vi "Actor Core.vi"(8 "error in":errorcluster, 11 "Assert Display in":refnum<class "Assert Display.lvclass">) -> (0 "error out":errorcluster, 3 "Actor out":refnum<class "Actor.lvclass">)   [LabVIEW 2016, in "Assert Display.lvlib" / "Assert Display.lvclass"]
doc: "(<B>Filename</B>: Actor Framework.lvlib:Actor.lvclass:Actor Core.vi)\n\nReceives messages to the actor, reacts to them, and initiates any error handling that may shut the actor down.\n\nDescendant classes may override this VI to append parallel tasks for the actor to complete while it handles messages. Overrides use the Call Parent Method node."
uses:
  Assert Display.lvclass
  C:/Program Files (x86)/National Instruments/LabVIEW 2016/vi.lib/ActorFramework/Actor/Actor.lvclass
  D:/Work/Projects/Actor_Assert_API/Base UI Actor/Base UI Actor/Base UI Actor.lvclass
  <vilib>/ActorFramework/Actor/Actor.lvclass
  Filter Config Display/Filter Config Display/Filter Config Display.lvclass
  D:/Work/Projects/Actor_Assert_API/Base UI Component/Base UI Component/Base UI Component.lvclass
  Main Display/Main Display/Main Display.lvclass
  Service Config Display/Service Config Display/Service Config Display.lvclass
  Base UI Actor/Base UI Actor/Base UI Actor.lvclass/Base UI Actor.ctl
  <vilib>/ActorFramework/Actor/Actor.lvclass/Actor.ctl
  <vilib>/ActorFramework/Message Enqueuer/Message Enqueuer.lvclass/Message Enqueuer.ctl
  Assert Display.lvclass/Assert Display.ctl
  Assert Display Messages/Change Screen Msg/Change Screen Msg.lvclass/Change Screen Msg.ctl
  <vilib>/ActorFramework/Message Enqueuer/Init from Existing Queue.vi
  <vilib>/ActorFramework/Message Enqueuer/Enqueue.vi
  <vilib>/ActorFramework/Stop Msg/Stop Msg.lvclass
  C:/Program Files (x86)/National Instruments/LabVIEW 2016/vi.lib/ActorFramework/Message/Message.lvclass
  Assert Display Messages/Change Screen Msg/Change Screen Msg.lvclass
  <vilib>/ActorFramework/Message Priority Queue/Priority Enqueue.vi
  <vilib>/ActorFramework/Message Enqueuer/Message Enqueuer.lvclass
  Base UI Actor/Base UI Actor/Base UI Actor.lvclass
  Base UI Component/Base UI Component/Base UI Component.lvclass
panel:
  in  "Filters":bool
  in  "Services":bool
  in  "Main":bool
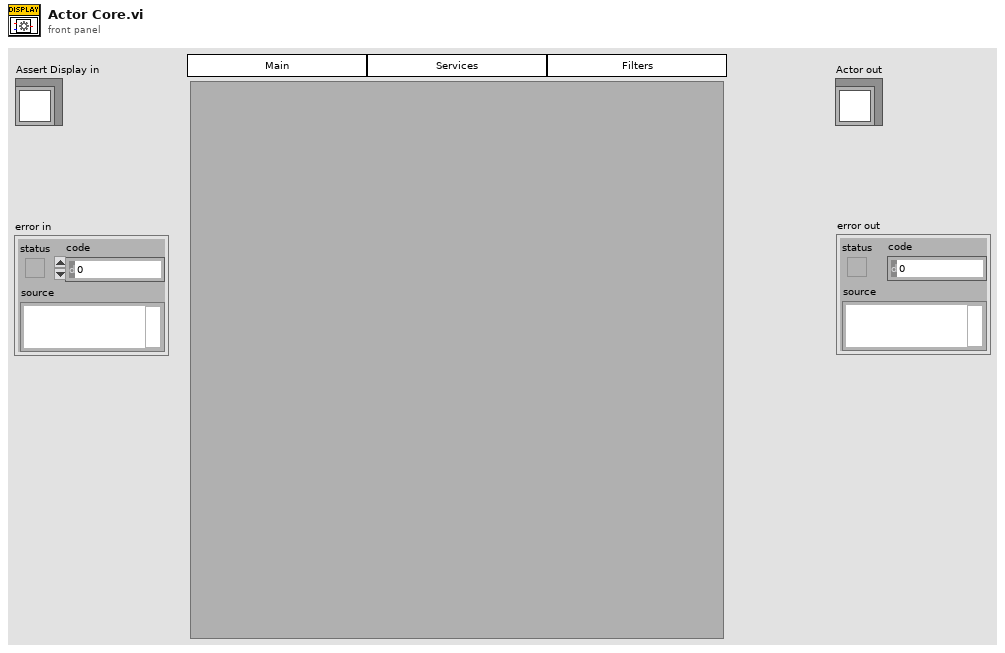
[diagram p1: front panel]
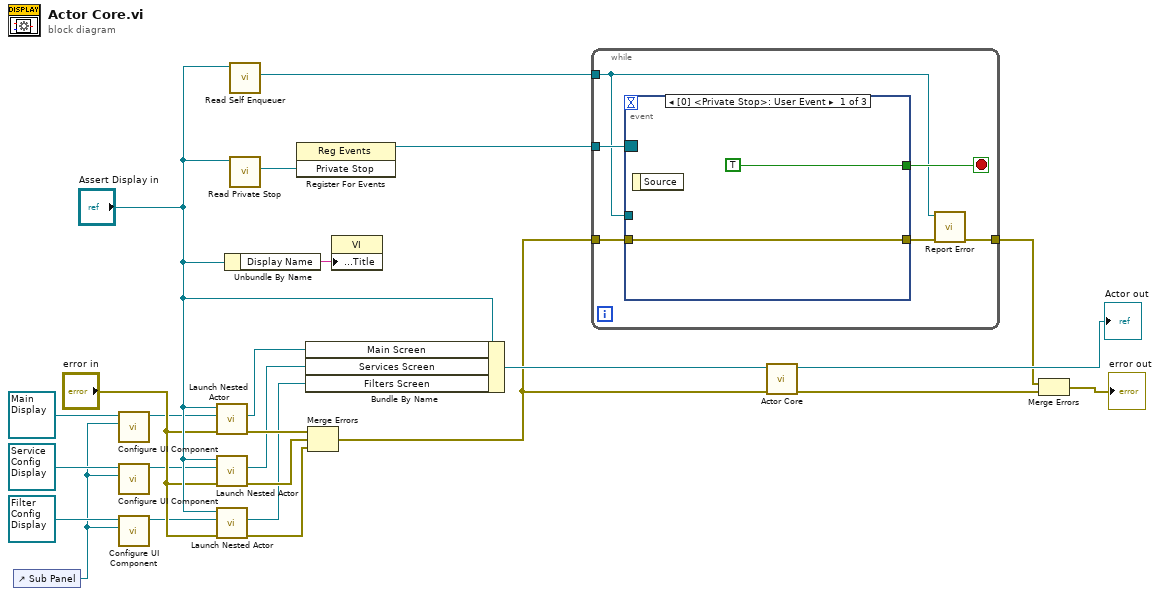
[diagram p0: block diagram]
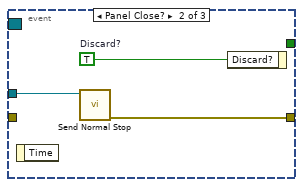
[diagram p2: hidden frame]
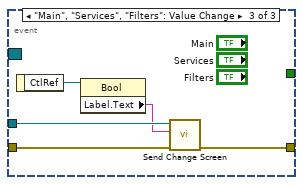
[diagram p3: hidden frame]
diagram:
  n1 = control-ref of="Sub Panel"() -> (w1:refnum<vi>)
  n2 = call "Configure UI Component.vi"("SubPanel Reference"=w1, "Base UI Component in"=refnum<class "Main Display.lvclass"> refnum ("Assert Display.lvlib:Main Display.lvlib:Main Display.lvclass")) -> ("Base UI Component out"=w4:refnum<class "Main Display.lvclass">)  [unwired: 9 in]
  n3 = call "Configure UI Component.vi"("SubPanel Reference"=w1, "Base UI Component in"=refnum<class "Service Config Display.lvclass"> refnum ("Assert Display.lvlib:Service Config Display.lvlib:Service Config Display.lvclass")) -> ("Base UI Component out"=w3:refnum<class "Service Config Display.lvclass">)  [unwired: 9 in]
  n4 = call "Configure UI Component.vi"("SubPanel Reference"=w1, "Base UI Component in"=refnum<class "Filter Config Display.lvclass"> refnum ("Assert Display.lvlib:Filter Config Display.lvlib:Filter Config Display.lvclass")) -> ("Base UI Component out"=w2:refnum<class "Filter Config Display.lvclass">)  [unwired: 9 in]
  n5 = call <vilib>:"Launch Nested Actor.vi"("error in (no error)"="error in", "Nested Actor"=w4, "Caller Actor in"="Assert Display in") -> ("error out"=w14:errorcluster, "Nested Actor's Enqueuer"=w10:refnum<class "Message Enqueuer.lvclass">)  [unwired: 6 in, 1 out]
  n6 = call <vilib>:"Launch Nested Actor.vi"("error in (no error)"="error in", "Nested Actor"=w3, "Caller Actor in"="Assert Display in") -> ("error out"=w13:errorcluster, "Nested Actor's Enqueuer"=w9:refnum<class "Message Enqueuer.lvclass">)  [unwired: 6 in, 1 out]
  n7 = call <vilib>:"Launch Nested Actor.vi"("error in (no error)"="error in", "Nested Actor"=w2, "Caller Actor in"="Assert Display in") -> ("error out"=w12:errorcluster, "Nested Actor's Enqueuer"=w8:refnum<class "Message Enqueuer.lvclass">)  [unwired: 6 in, 1 out]
  n8 = Unbundle By Name("Assert Display in") -> ("Display Name"=w23:string)
  n9 = call <vilib>:"Read Self Enqueuer.vi"("Actor"="Assert Display in") -> ("Self Enqueuer"=w20:refnum<class "Message Enqueuer.lvclass">)  [unwired: 10 in]
  n10 = call "Read Private Stop.vi"("Base UI Actor in"="Assert Display in") -> ("Private Stop"=w22:refnum<user-event>)  [unwired: 10 in]
  n11 = register-events(w22) -> (reference out=w21:refnum<event-registration>)  [unwired: 2 in, 1 out]
  n12 = Bundle By Name(cluster="Assert Display in", "Main Screen"=w10, "Services Screen"=w9, "Filters Screen"=w8) -> (w11:refnum<class "Assert Display.lvclass">)
  n13 = Merge Errors(w14, w13, w12) -> (w7:errorcluster)
  n14 = property class="VI"("Front Panel.Title"=w23) -> ()  [unwired: 2 in, 2 out]
  n15 = while {
    tunnel: w21 -> [w31]
    tunnel: w20 -> [w26]
    tunnel: w7 -> [w29]
    tunnel: [w27] -> w5
    stop <- w30 stop-if-true
    n16 = event shown="[0] <Private Stop>: User Event" {
      selector: w31 -> [_ _ _]
      dyn-events: _ -> [_ _ _]
      timeout: _ -> [_ _ _]
      tunnel: [TRUE _ _] -> w30
      tunnel: w26 -> [_ w35 w41]
      tunnel: w29 -> [w32 _ w38]
      tunnel: [w32 w34 w37] -> w28
      event User Event {
        n17 = event-data() -> ()  [unwired: 1 in, 1 out]
      }
      event Panel Close? {
        w36 = TRUE  # Discard?
        n18 = event-data() -> ()  [unwired: 1 in, 1 out]
        n19 = call <vilib>:"Send Normal Stop.vi"("Message Enqueuer"=w35) -> ("error out"=w34:errorcluster)  [unwired: 10 in]
        n20 = event-data("Discard?"=w36) -> ()  [unwired: 1 in, 1 out]
      }
      event "Main", "Services", "Filters": Value Change {
        n21 = event-data() -> ("CtlRef"=w40:refnum<vi>)  [unwired: 1 in]
        n22 = property class="Bool"(reference=w40) -> ("Label.Text"=w39:string)  [unwired: 1 in, 2 out]
        n23 = call "Send Change Screen.vi"("error in (no error)"=w38, "Screen"=w39, "Message Enqueuer"=w41) -> ("error out"=w37:errorcluster)  [unwired: 7 in, 1 out]
      }
    }
    n24 = call "Report Error.vi"("error in (no error)"=w28, "Self Enqueuer"=w26) -> ("error out"=w27:errorcluster)  [unwired: 9 in]
  }
  n25 = call-parent "Actor Core.vi"("error in"=w7, "Actor in"=w11) -> ("error out"=w25:errorcluster, "Actor out"=→"Actor out":refnum<class "Actor.lvclass">)  [unwired: 8 in]
  n26 = Merge Errors(w5, w25) -> (→"error out":errorcluster)
